vi "Execute.vi"(5 "Init user event out":refnum<user-event>, 7 "user event in":refnum<user-event>, 8 "Advanced Waveform In":refnum<class "Advanced Waveform.lvclass">, 9 "Display Message in":refnum<class "Display Message.lvclass">, 10 "Command Queue":refnum<queue>, 11 "error in (no error)":errorcluster) -> (0 "Advanced Waveform Out":refnum<class "Advanced Waveform.lvclass">, 1 "Display Message out":refnum<class "Display Message.lvclass">, 2 "Stop":bool, 3 "error out":errorcluster)   [LabVIEW 2011, in "Display Message.lvclass"]
uses:
  Display Message.lvclass
  Advanced Waveform Class/Advanced Waveform.lvclass
  Message.lvclass
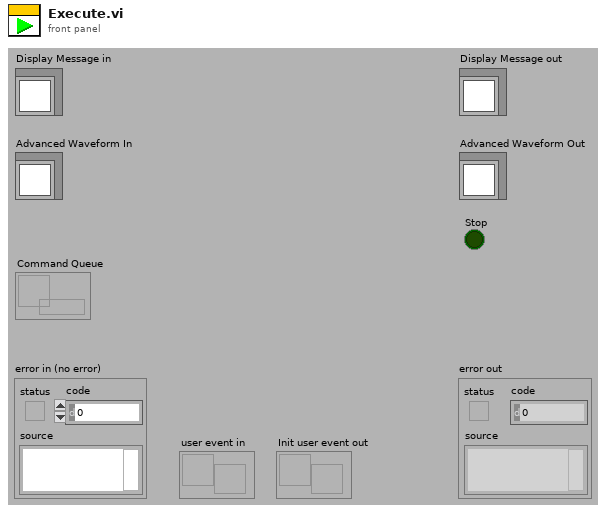
[diagram p1: front panel]
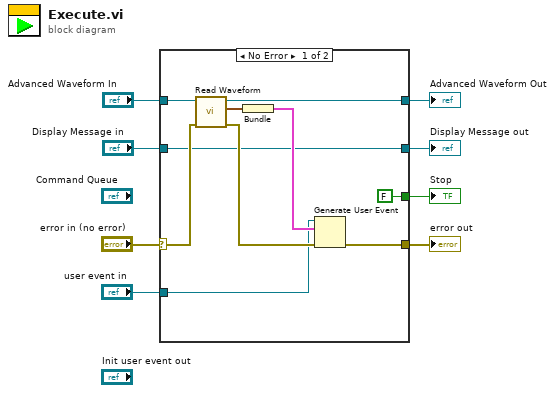
[diagram p0: block diagram]
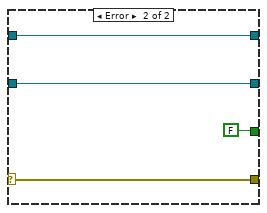
[diagram p2: hidden frame]
diagram:
  n1 = case shown="No Error" "error in (no error)" {
    selector: "error in (no error)" -> [w17 w22]
    tunnel: [w12 w22] -> w7
    tunnel: [FALSE FALSE] -> w6
    tunnel: "Display Message in" -> [w9 w20]
    tunnel: [w9 w20] -> w4
    tunnel: [w14 w19] -> w3
    tunnel: "Advanced Waveform In" -> [w18 w19]
    tunnel: "user event in" -> [w11 _]
    frame No Error {
      n2 = call-dynamic "Read Waveform.vi"("error in (no error)"=w17, "Waveform in"=w18) -> ("error out"=w13:errorcluster, "Waveform"=w15:waveform(dbl), "Waveform out"=w14:refnum<class "Advanced Waveform.lvclass">)  [unwired: 7 in]
      n3 = Bundle("Waveform"=w15) -> (w16:cluster{"Waveform":waveform(dbl)})  [unwired: 1 in]
      n4 = Generate User Event(user event=w11, event data cluster=w16, error in=w13) -> (error out=w12:errorcluster)  [unwired: 1 out]
    }
    frame Error {
    }
  }
  "error out" <- w7
  "Display Message out" <- w4
  "Stop" <- w6
  "Advanced Waveform Out" <- w3
